vi "GetPluginPath.vi"(8 "error in (no error)":errorcluster, 10 "Base Path":path=path "../../MyPlugins/Keysight335XX/Keysight335XX.ini", 11 "Path to Plugin INI\n(complete)":path=path "../../MyPlugins/Keysight335XX/Keysight335XX.ini") -> (0 "error out":errorcluster, 3 "Path to Class":path=path "../../MyPlugins/Keysight335XX/Keysight335XX.ini")   [LabVIEW 2014, in "FGenPlugins.lvlib" / "NISTFGenPluginsBase.lvclass"]
uses:
  NISTFGenPluginsBase.lvclass
  <userlib>/NIST/BaseClasses/Object_class/BaseObject.lvclass
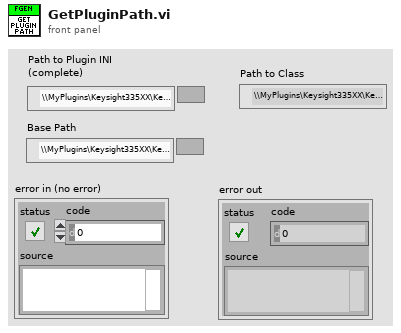
[diagram p1: front panel]
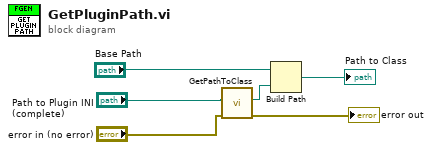
[diagram p0: block diagram]
diagram:
  n1 = call <userlib>:"GetPathToClass.vi"("error in (no error)"="error in (no error)", "configuration file path"="Path to Plugin INI\n(complete)") -> ("error IO"=→"error out":errorcluster, "PathToClass"=w6:path)  [unwired: 8 in]
  n2 = Build Path(base path="Base Path", name or relative path=w6) -> (appended path=→"Path to Class":path)
